vi "test Get Parameters.vi"(8 "error in":errorcluster, 11 "TestCase in":refnum<class "Scripting.lvclass">) -> (0 "error out":errorcluster, 3 "TestCase out":refnum<class "Scripting.lvclass">)   [LabVIEW 2020, in "Scripting.lvclass"]
uses:
  Scripting.lvclass
  Shared/Parameter Definition.ctl
  Encoding and Decoding/Encoding.ctl
  Scripting.lvclass/Scripting.ctl
  Scripting/Constants.vi
  <vilib>/NI VeriStand/Custom Device Tools/Custom Device Utility Library/NI VeriStand - Search for Item by GUID.vi
  <vilib>/addons/_JKI Toolkits/VI Tester/TestCase.llb/TestCase.lvclass
  Scripting/Communication Bus Template Scripting.lvlib
  Encoding and Decoding/Encoding and Decoding.lvlib
  <vilib>/NI VeriStand/Custom Device Tools/Custom Device Utility Library/Custom Device Utility Library.lvlib
  C:/Program Files (x86)/National Instruments/LabVIEW 2020/vi.lib/addons/_JKI Toolkits/VI Tester/TestCase.llb/TestCase.lvclass
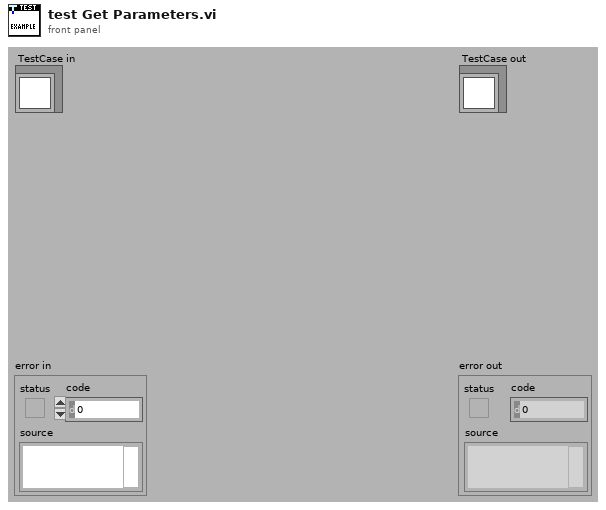
[diagram p1: front panel]
types:
  T1 = typedef "Parameter Definition.ctl" = cluster{"start index":i32, "size":i32, "encoding":T2, "signed":bool, "scale multiplier":dbl, "scale offset":dbl}
  T2 = typedef "Encoding and Decoding.lvlib/Encoding.ctl" = enum16{"BNR", "BCD", "Discrete"}
  T3 = typedef "Custom Device API.lvlib/Custom Device Item Ref.ctl" = u64
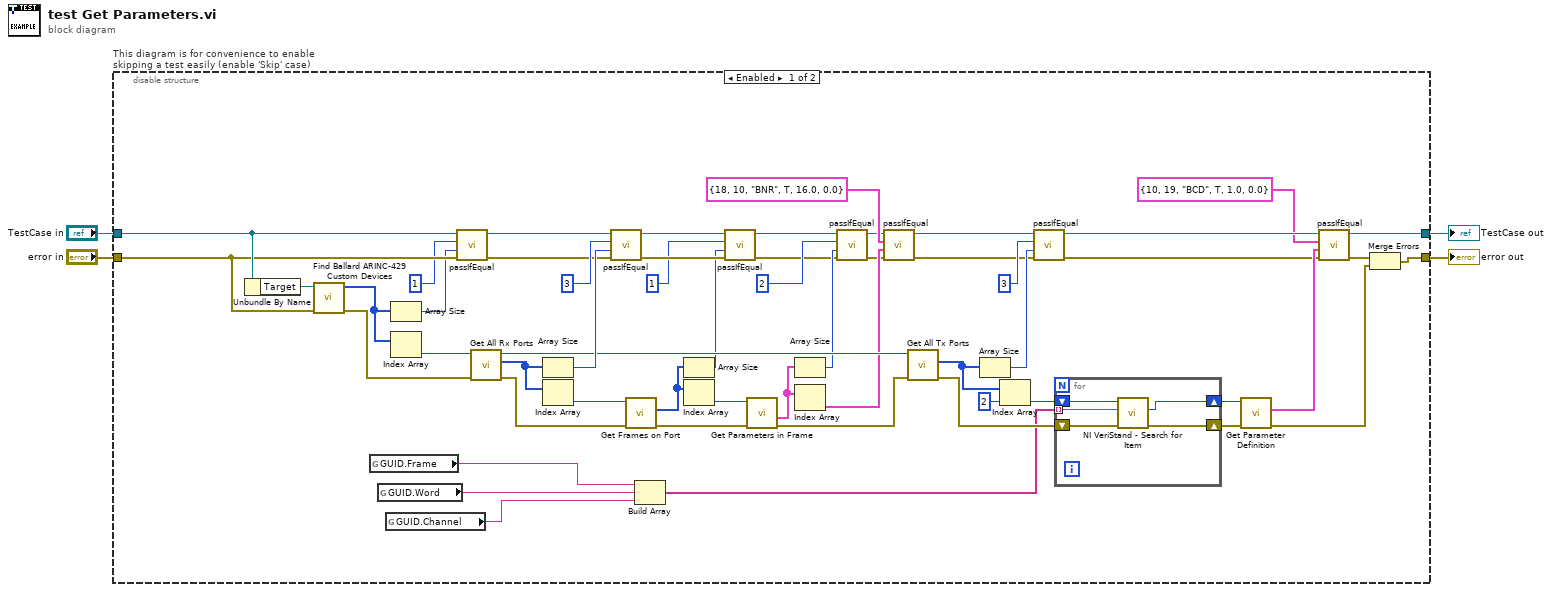
[diagram p0: block diagram]
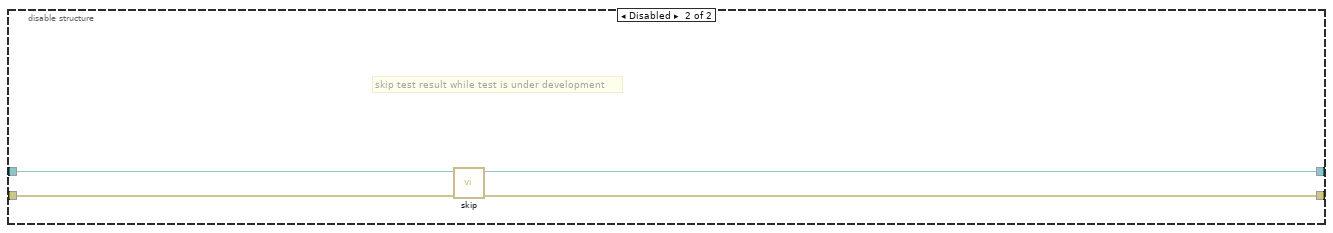
[diagram p2: hidden frame]
diagram:
  n1 = disable-structure "This diagram is for convenience to enable skipping a test easily (enable 'Skip' case)" shown="Enabled" {
    disable-tunnel: "TestCase in" -> [w56 w68]
    disable-tunnel: [w29 w66] -> w1
    disable-tunnel: [w37 w67] -> w3
    disable-tunnel: "error in" -> [w55 w65]
    frame Enabled {
      n2 = Unbundle By Name(w56) -> ("Target"=w58:refnum<k24>)
      n3 = call "Find Ballard ARINC-429 Custom Devices.vi"("error in"=w55, "target"=w58) -> ("error out"=w46:errorcluster, "Ballard ARINC-429 custom devices"=w54:u64[])  [unwired: 8 in]
      n4 = global read "Constants.vi" "GUID.Frame"() -> (w12:string)
      n5 = global read "Constants.vi" "GUID.Word"() -> (w11:string)
      n6 = global read "Constants.vi" "GUID.Channel"() -> (w10:string)
      n7 = Array Size(array=w54) -> (size(s)=w52:i32)
      n8 = Index Array(array=w54) -> (element=w57:u64)  [unwired: 1 in]
      n9 = call-dynamic "passIfEqual.vi"("error in (no error)"=w55, "y"=w52, "x"=1 ("size(s)"), "TestCase in"=w56) -> ("error out"=w47:errorcluster, "TestCase out"=w48:refnum<class "Scripting.lvclass">)  [unwired: 6 in]
      n10 = call "Get All Rx Ports.vi"("error in"=w46, "Ballard ARINC 429 custom device in"=w57) -> ("error out"=w6:errorcluster, "Rx hardware channel refs"=w51:T3[], "Ballard ARINC 429 custom device out"=w45:T3)  [unwired: 7 in]
      n11 = Array Size(array=w51) -> (size(s)=w49:i32)
      n12 = Index Array(array=w51) -> (element=w8:T3)  [unwired: 1 in]
      n13 = call-dynamic "passIfEqual.vi"("error in (no error)"=w47, "y"=w49, "x"=3 ("size(s)"), "TestCase in"=w48) -> ("error out"=w23:errorcluster, "TestCase out"=w24:refnum<class "Scripting.lvclass">)  [unwired: 6 in]
      n14 = call "Get Frames on Port.vi"("error in"=w6, "port ref in"=w8) -> ("error out"=w5:errorcluster, "frame references"=w7:T3[])  [unwired: 6 in, 2 out]
      n15 = Build Array(w12, w11, w10) -> (w9:string[])
      n16 = Array Size(array=w7) -> (size(s)=w20:i32)
      n17 = Index Array(array=w7) -> (element=w22:T3)  [unwired: 1 in]
      n18 = call-dynamic "passIfEqual.vi"("error in (no error)"=w23, "y"=w20, "x"=1 ("size(s)"), "TestCase in"=w24) -> ("error out"=w15:errorcluster, "TestCase out"=w16:refnum<class "Scripting.lvclass">)  [unwired: 6 in]
      n19 = call "Get Parameters in Frame.vi"("error in"=w5, "frame ref in"=w22) -> ("error out"=w26:errorcluster, "parameter definitions"=w19:T1[])  [unwired: 6 in, 2 out]
      n20 = Array Size(array=w19) -> (size(s)=w17:i32)
      n21 = Index Array(array=w19) -> (element=w25:T1)  [unwired: 1 in]
      n22 = call-dynamic "passIfEqual.vi"("error in (no error)"=w15, "y"=w17, "x"=2 ("size(s)"), "TestCase in"=w16) -> ("error out"=w13:errorcluster, "TestCase out"=w14:refnum<class "Scripting.lvclass">)  [unwired: 6 in]
      n23 = call-dynamic "passIfEqual.vi"("error in (no error)"=w13, "y"=w25, "x"=T1 {"start index"=18, "size"=10, "encoding"=enum."BNR", "signed"=TRUE, "scale multiplier"=16.0, "scale offset"=0.0} ("parameter definition"), "TestCase in"=w14) -> ("error out"=w41:errorcluster, "TestCase out"=w42:refnum<class "Scripting.lvclass">)  [unwired: 6 in]
      n24 = call "Get All Tx Ports.vi"("error in"=w26, "Ballard ARINC 429 custom device in"=w45) -> ("error out"=w35:errorcluster, "Tx hardware channel refs"=w40:T3[])  [unwired: 7 in, 1 out]
      n25 = Array Size(array=w40) -> (size(s)=w43:i32)
      n26 = Index Array(array=w40, index=2) -> (element=w36:T3)
      n27 = call-dynamic "passIfEqual.vi"("error in (no error)"=w41, "y"=w43, "x"=3 ("size(s)"), "TestCase in"=w42) -> ("error out"=w31:errorcluster, "TestCase out"=w30:refnum<class "Scripting.lvclass">)  [unwired: 6 in]
      n28 = for {
        tunnel: w9 -> [w60] mode=indexing
        shift-right: [w61] -> w33
        shift-left: w36 -> [w64]
        shift-right: [w62] -> w34
        shift-left: w35 -> [w63]
        n29 = call-poly <vilib>:"NI VeriStand - Search for Item.vi"("error in"=w63, "Item GUID"=w60, "Section Ref in"=w64) -> ("error out"=w62:errorcluster, "Item Ref"=w61:T3)  [unwired: 5 in, 2 out]
      }
      n30 = call "Get Parameter Definition.vi"("error in"=w34, "parameter ref in"=w33) -> ("error out"=w38:errorcluster, "parameter definition"=w32:T1)  [unwired: 7 in, 1 out]
      n31 = call-dynamic "passIfEqual.vi"("error in (no error)"=w31, "y"=w32, "x"=T1 {"start index"=10, "size"=19, "encoding"=enum."BCD", "signed"=TRUE, "scale multiplier"=1.0, "scale offset"=0.0} ("parameter definition"), "TestCase in"=w30) -> ("error out"=w28:errorcluster, "TestCase out"=w29:refnum<class "Scripting.lvclass">)  [unwired: 6 in]
      n32 = Merge Errors(w28, w38) -> (w37:errorcluster)
    }
    frame Disabled {
      # "skip test result while test is under development"
      n33 = call <vilib>:"skip.vi"("error in (no error)"=w65, "TestCase in"=w68) -> ("error out"=w67:errorcluster, "TestCase out"=w66:refnum<class "Scripting.lvclass">)  [unwired: 8 in]
    }
  }
  "error out" <- w3
  "TestCase out" <- w1
